vi "Deadzone.vi"(1 "Deadzone":dbl, 2 "Input":dbl) -> (0 "Output":dbl)   [LabVIEW 2012]
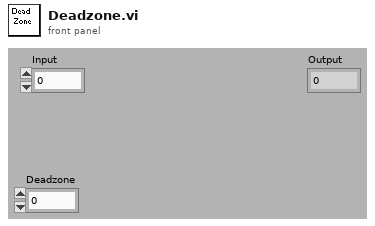
[diagram p1: front panel]
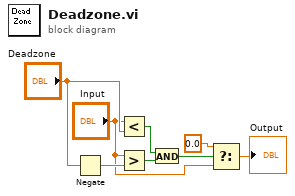
[diagram p0: block diagram]
diagram:
  n1 = Negate(x="Deadzone") -> (-x=w8:dbl)
  n2 = Less?(x="Input", y="Deadzone") -> (x < y?=w6:bool)
  n3 = Greater?(x="Input", y=w8) -> (0:w5:bool)
  n4 = And(x=w6, y=w5) -> (x .and. y?=w4:bool)
  n5 = Select(t=0.0, s=w4, f="Input") -> (s? t:f=→"Output":dbl)
